vi "GUI_visable_ctr (SubVI).vi"(8 "error out 2":errorcluster, 10 "Array":refnum<vi>[](array[refnum]), 11 "Visible":bool) -> (0 "error out":errorcluster)   [LabVIEW 2017]
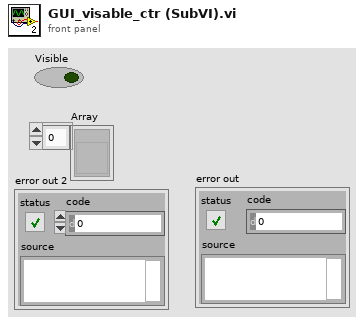
[diagram p1: front panel]
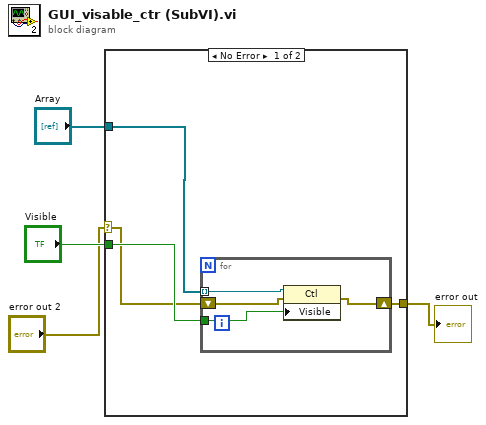
[diagram p0: block diagram]
diagram:
  n1 = case shown="No Error" "error out 2" {
    selector: "error out 2" -> [w5 w13]
    tunnel: "Visible" -> [w8 _]
    tunnel: "Array" -> [w7 _]
    tunnel: [w6 w13] -> w2
    frame No Error {
      n2 = for {
        tunnel: w7 -> [w12] mode=indexing
        tunnel: w8 -> [w9]
        shift-right: [w11] -> w6
        shift-left: w5 -> [w10]
        n3 = property class="Ctl"(reference=w12, error in=w10, "Visible"=w9) -> (error out=w11:errorcluster)  [unwired: 1 out]
      }
    }
    frame Error {
    }
  }
  "error out" <- w2
